vi "扫描文件.vi"() -> ()   [LabVIEW 2010]
panel:
  out "输出字符":string
  out "输出数字":dbl
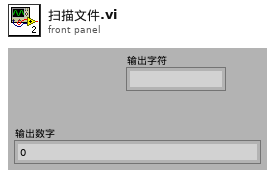
[diagram p1: front panel]
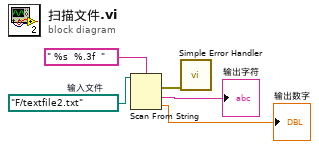
[diagram p0: block diagram]
diagram:
  w5 = path "F:/textfile2.txt"  # 输入文件
  n1 = Scan From String(" %s  %.3f  " ("格式字符串"), w5) -> (w3:errorcluster, output 1=→"输出字符":string, output 2=→"输出数字":dbl)  [unwired: 3 in, 1 out]
  n2 = call <vilib>:"Simple Error Handler.vi"("error in (no error)"=w3) -> ()  [unwired: 4 in, 5 out]
